vi "Einzelne Stufe aendern.vi"(4 "Component additional Index":i32[](array[numeric]), 5 "GD-Cluster":T3, 6 "Component GD Index":i32[](array[numeric]), 7 "GD LNI Cluster":T2, 8 "error in (no error)":errorcluster caption="Fehler (Eingang, kein Fehler)", 9 "Komponentenauswahl":T7 {"Konzentration" format="%#.6f"}, 10 "Zeile Punkt Änderung Cluster":cluster{"Zeile":i32, "Punkt":string}, 11 "Stufen Tabellen in":string[][][](array[string])) -> (0 "error out":errorcluster caption="Fehler (Ausgang)", 1 "Component Index out":i32, 2 "Komponente out":T6, 3 "GD out":T5)   [LabVIEW 2020, in "Linearisierung v2.lvlib" / "Gasteiler.lvlib"]
uses:
  Gasteiler.lvlib
  KomponentenArray.ctl
  Visualisierungs Elemente/Auswahlfeld.ctl
  Seiten/System Einstellungen V2/Traegergas.ctl
  Visualisierungs Elemente/Checkbox(boolsch).ctl
  Aktionen FGV Gasteiler Daten.ctl
  Aktion FGV Gasteilerliste laden.ctl
  AK-Komm Gasteiler/Aktionen AK Komm.ctl
  AK-Komm Gasteiler/Alter Gasteiler/Aktionen AK Komm_ALT.ctl
  Horiba/Aktion Befehl.ctl
  AK-Komm Gasteiler/AK Komm Gasteiler.lvlib
  Horiba/Horiba GDC.lvlib
  AK-Komm Gasteiler/Alter Gasteiler/Alter Gasteiler.lvlib
  Linearisierung v2.lvlib
  Aktion Lin Daten aufarbeiten.ctl
  Seiten/System Einstellungen V2/System Einstellungen V2.lvlib
  HovaCal/HovaCal.lvlib
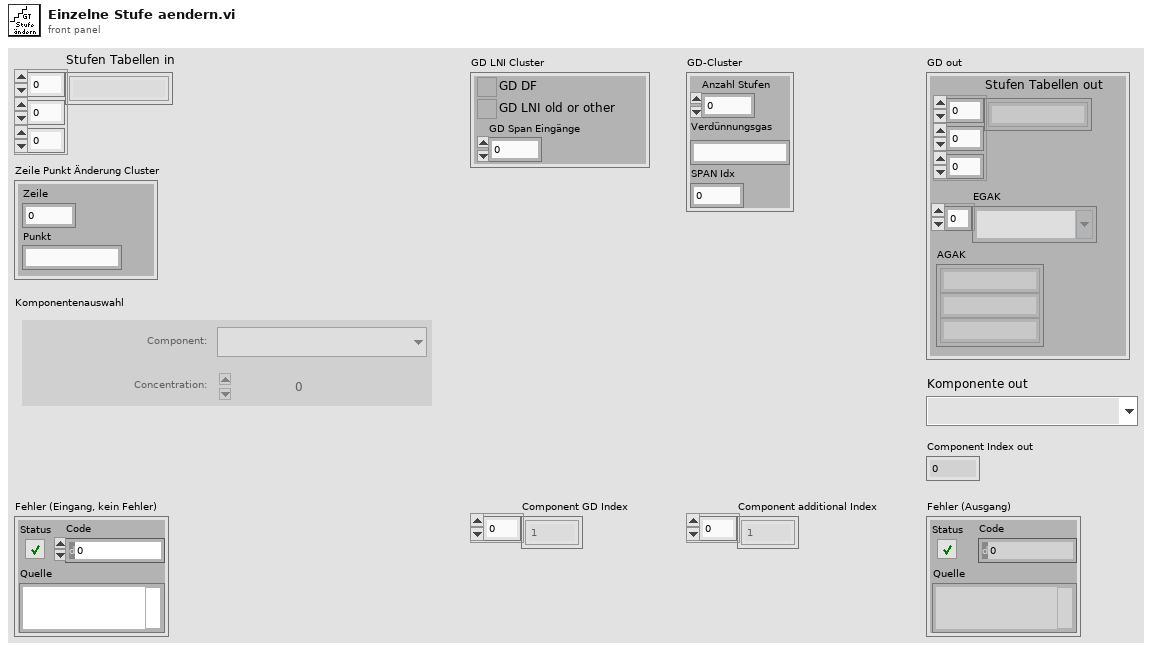
[diagram p1: front panel]
types:
  T1 = typedef "Checkbox(boolsch).ctl" = bool
  T2 = cluster{"GD DF":T1, "GD LNI old or other":T1, "GD Span Eingänge":u16}
  T3 = cluster{"Anzahl Stufen":sgl, "Verdünnungsgas":string, "SPAN Idx":i32}
  T4 = typedef "System Einstellungen V2.lvlib/Traegergas.ctl" = string
  T5 = cluster{"Stufen Tabellen out":string[][][], "EGAK":T4[], "AGAK":string[]}
  T6 = typedef "Auswahlfeld.ctl" = u16
  T7 = typedef "Linearisierung v2.lvlib/KomponentenArray.ctl" = cluster{"Komponente:":T6, "Konzentration":dbl}[]
  T8 = typedef "Linearisierung v2.lvlib/Gasteiler.lvlib/Aktionen FGV Gasteiler Daten.ctl" = enum16{"lesen", "Gasteiler Daten", "Seriellen Param.", "MB-Endwert", "laden", "speichern", "Anforderung", "TCP", "Aufzeichnung Start"}
  T9 = typedef "Linearisierung v2.lvlib/Aktion Lin Daten aufarbeiten.ctl" = enum16{"lesen", "Protkolldaten", "speichern", "laden", "EPA auswerten", "Tabelle schreiben", "Lin auswerten", "Tab init", "Stufentabelle", "EPA aktiviert", "Nachbehandlung laden", "Tabelle löschen", "Istwerte löschen", "Zeile löschen", "Zeile einfügen", "LIN aktiviert", "LIN/EPA aktiv laden", "EGAK Tab", "LIN übernehmen", "Tab init ohne Stufen"}
  T10 = typedef "Linearisierung v2.lvlib/Lin-Polynom Daten.ctl" = cluster{"Messgerät":string, "Kalibrator (Gasteiler)":string, "Bearbeiter/in":string, "Komponente":string, "Zeitstempel":timestamp, "F_max gefordert (%)":sgl, "F_max in %":sgl, "F_max in ppm":sgl, "Vorschlag Ordnung":i32, "Polynom OK":bool, "Polynomkoeff.":dbl[], "Prüfgas Konzentration":dbl, "Pfad EPA":string, "Pfad_LIN":string, "Gasnummer:":u8, "Komponentenauswahl":T7, "Verdünnungsgas":T11, "Zeitdauer Stufe":T12, "Anzahl Stufen":T12, "F_max in % EPA":sgl, "F_max in ppm EPA":sgl, "F_max in % LIN":sgl, "F_max in ppm LIN":sgl, "Punkte umkehren":bool, "EPA Optionsfeld":T13, "Autolin Hovacal":T14, "Spanfactors":sgl[], "Kalibrierauswahl":T15, "Conditions:":T16, "Gasflaschen Nr.:":string, "Bottle Accuracy":dbl, "Konfig Gasflasche":T17, "Gasflasche":T18, "HovaCAL Flow AutoLin":T19, "MFC Output":T20, "Gas Ablaufdatum":timestamp, "Lin Modus":T21, "zusätzliche Zeitdauer Erster Punkt":sgl, "Offsets":sgl[]}
  T11 = typedef "Linearisierung v2.lvlib/Gasteiler.lvlib/Prüfgas in.ctl" = u16
  T12 = typedef "Zahlen-Eingabefeld.ctl" = sgl
  T13 = typedef "Linearisierung v2.lvlib/EPA Optionsfeld.ctl" = enum32{"Istwert", "Rohwert", "Linearisierter Wert"}
  T14 = typedef "Linearisierung v2.lvlib/Gasteiler.lvlib/HovaCal.lvlib/AutoLin Hovacal.ctl" = enum32{"Keine Auswahl", "Optionsauswahl 1", "Optionsauswahl 2"}
  T15 = typedef "Linearisierung v2.lvlib/Kalibrieroption.ctl" = u16
  T16 = typedef "Linearisierung v2.lvlib/Linearity verification 1065-307.lvlib/Condition.ctl" = u16
  T17 = typedef "System Einstellungen V2.lvlib/Konfig Gasflasche.ctl" = bool
  T18 = typedef "System Einstellungen V2.lvlib/Gasflasche Auswahl.ctl" = u16
  T19 = typedef "Linearisierung v2.lvlib/Gasteiler.lvlib/HovaCAL_Interface.lvlib/Controls.lvlib/Flow Einstellung.ctl" = cluster{"HovaCAL Flow Input Cluster":dbl}
  T20 = typedef "Linearisierung v2.lvlib/Gasteiler.lvlib/HovaCAL_Interface.lvlib/Controls.lvlib/Pump state.ctl" = cluster{"Run":bool}
  T21 = typedef "Linearisierung v2.lvlib/Lin Modus.ctl" = u16
  T22 = typedef "Linearisierung v2.lvlib/Gasteiler.lvlib/Aktion FGV Gasteilerliste laden.ctl" = enum16{"lesen", "laden", "speichern", "Liste erstellen", "Formel ändern", "Gas vereinzeln"}
  T23 = typedef "Linearisierung v2.lvlib/Gasteiler.lvlib/Gasteiler Daten.ctl" = cluster{"Gasteiler":T24, "Gasteiler Stufen":T25, "Gasteiler Type":T26, "Konfig Gasteiler":T27, "Gasteiler Span Eingänge":u16}
  T24 = typedef "String - Eingabefeld.ctl" = string
  T25 = typedef "Linearisierung v2.lvlib/Gasteiler.lvlib/Gasteiler Stufen.ctl" = u16
  T26 = typedef "Linearisierung v2.lvlib/GasteilerType.ctl" = u16
  T27 = typedef "System Einstellungen V2.lvlib/Gasteiler Auswahl.ctl" = u16
  T28 = typedef "Linearisierung v2.lvlib/Gasteiler.lvlib/AK Komm Gasteiler.lvlib/Aktionen AK Komm.ctl" = enum16{"lesen", "initialisieren", "beenden", "Status", "SMAN", "SREM", "STBY", "ASTF", "ASTZ", "SLST", "AGAT", "EGAK", "AGAK", "AKAK", "ADRU", "SKOP", "SVSA", "SVSZ", "SONO", "SAIR", "SNOX", "ANOX", "SSPL", "SRUC", "SLIN", "ALST", "ETYP", "SVIO", "LCYL", "CCYL", "DCYL", "SCYL", "GCYL", "DRGV", "DRDC"}
  T29 = typedef "Linearisierung v2.lvlib/Gasteiler.lvlib/AK Komm Gasteiler.lvlib/Alter Gasteiler.lvlib/Aktionen AK Komm_ALT.ctl" = enum16{"lesen", "initialisieren", "beenden", "SRES", "STBY", "SREM", "SMAN", "SLIN", "SLCH", "SLST", "SSPL", "AGAT", "ALST", "ASTZ", "ASTF", "AGAK", "EGAK"}
  T30 = typedef "Linearisierung v2.lvlib/Gasteiler.lvlib/Horiba GDC.lvlib/Aktion Befehl.ctl" = enum16{"lesen", "initialisieren", "Beenden", "Standby", "GD/CC", "Info", "Flow", "Alarm", "GD parameter", "GD point", "Durchfluss", "Spuelen1", "Spuelen1 On", "Spuelen1Off", "Spuelen2", "Ventil-Abfrage", "Reset"}
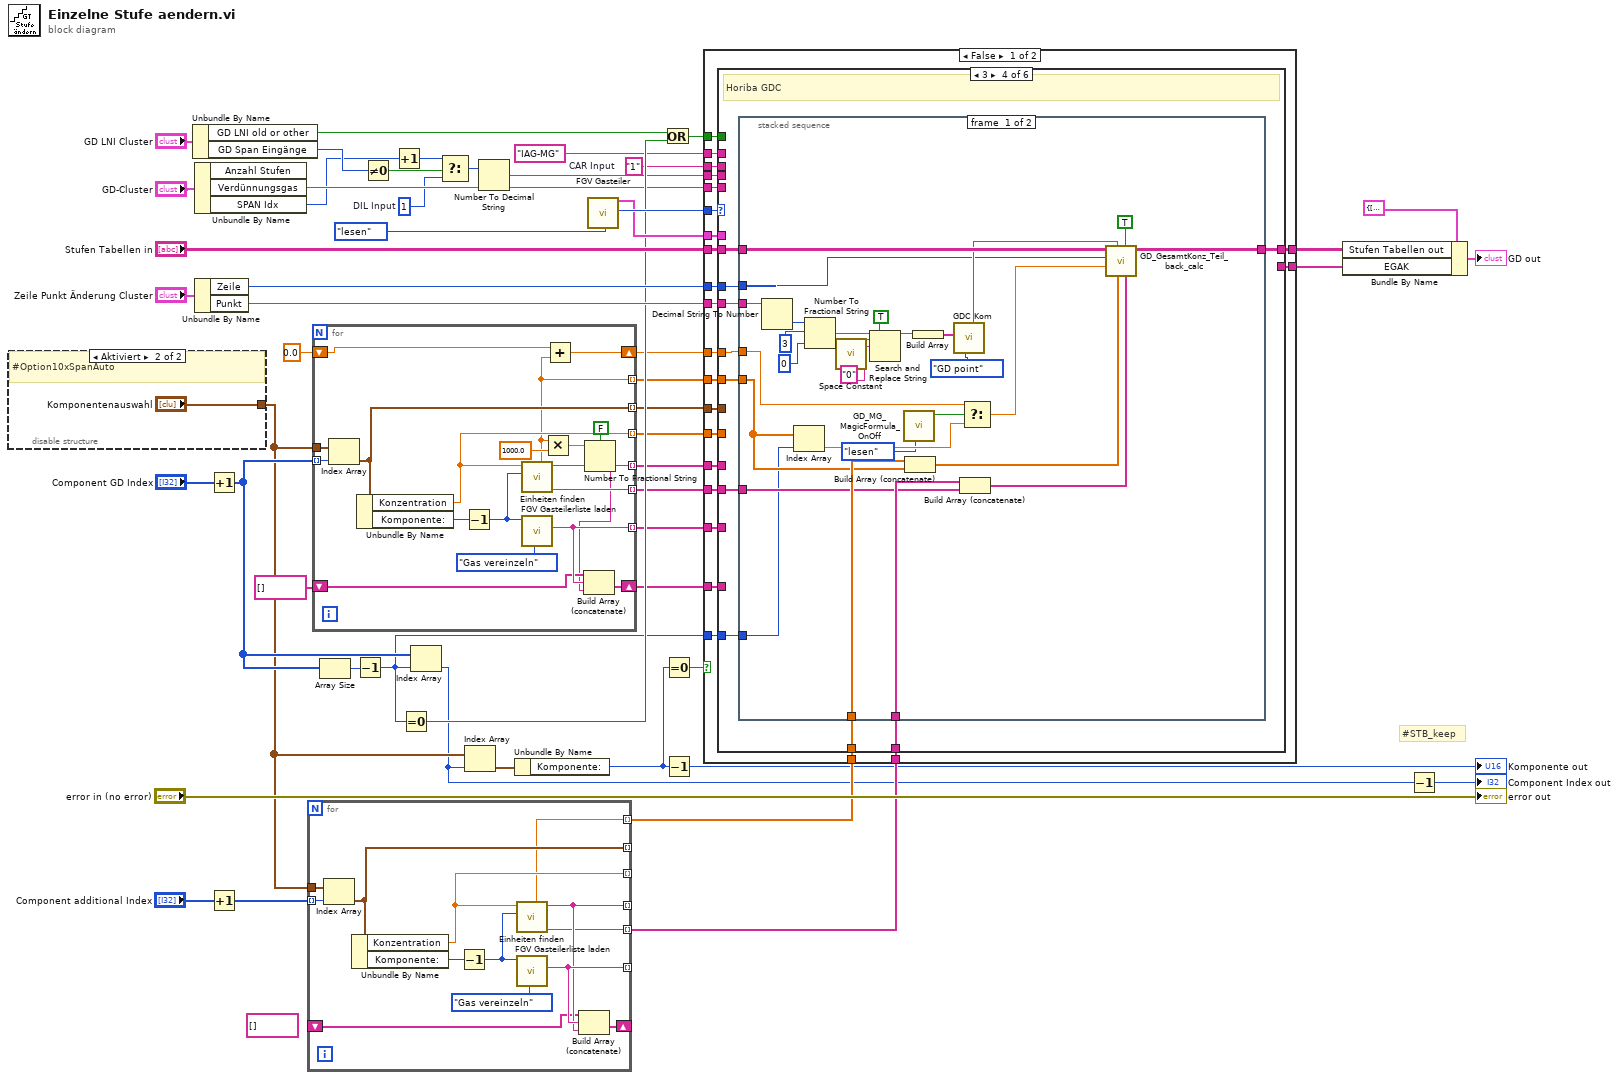
[diagram p0: block diagram]
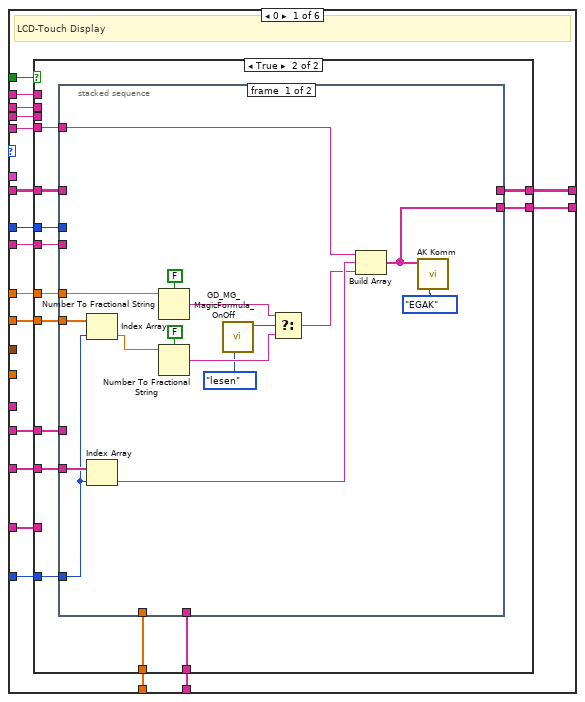
[diagram p2: hidden frame]
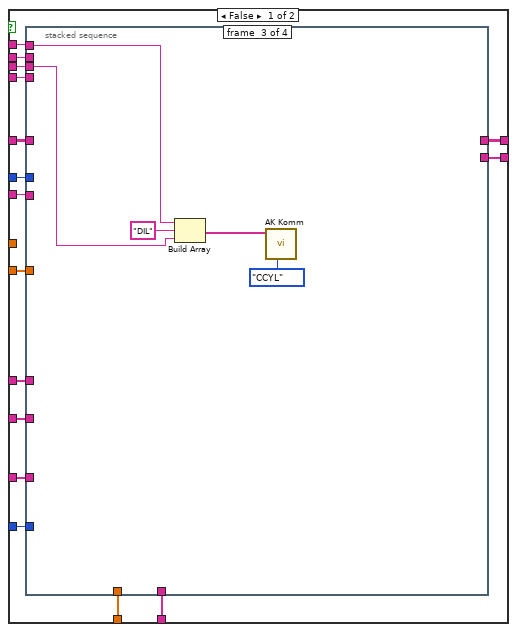
[diagram p3: hidden frame]
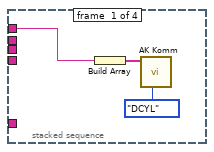
[diagram p4: hidden frame]
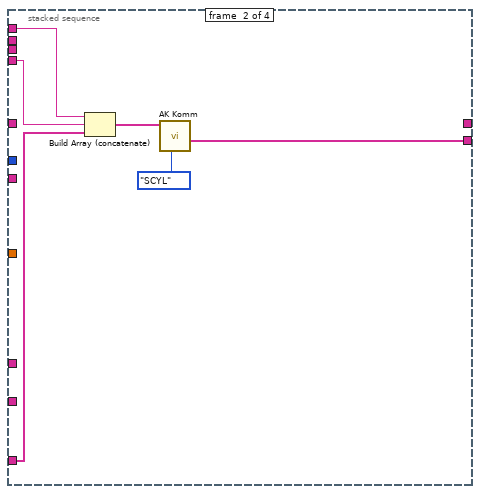
[diagram p5: hidden frame]
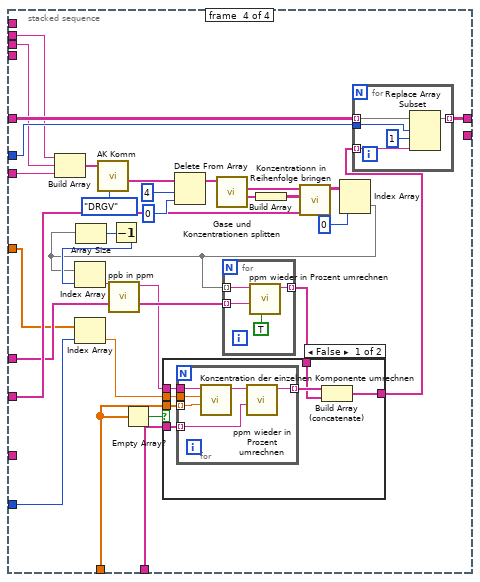
[diagram p6: hidden frame]
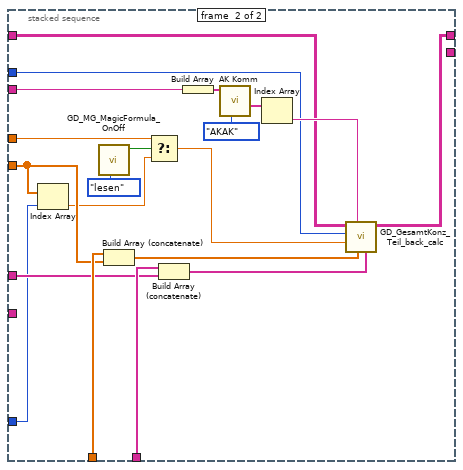
[diagram p8: hidden frame]
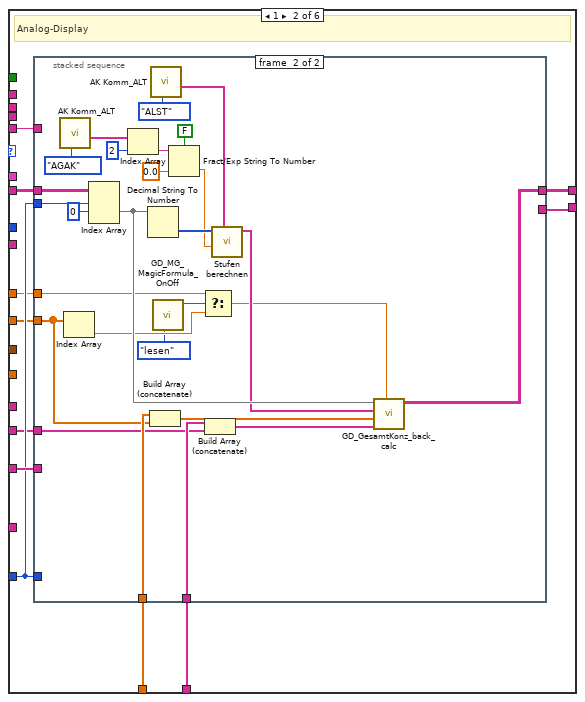
[diagram p9: hidden frame]
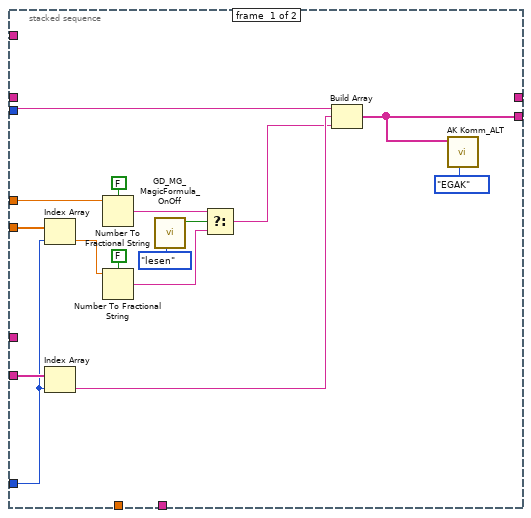
[diagram p10: hidden frame]
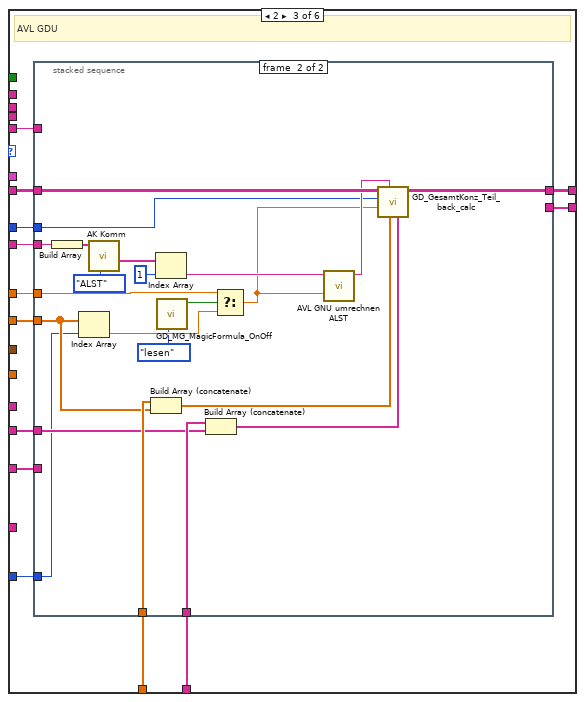
[diagram p11: hidden frame]
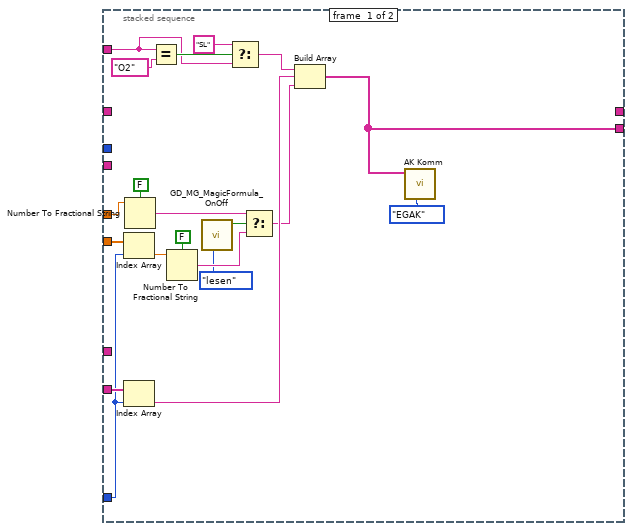
[diagram p12: hidden frame]
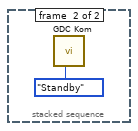
[diagram p13: hidden frame]
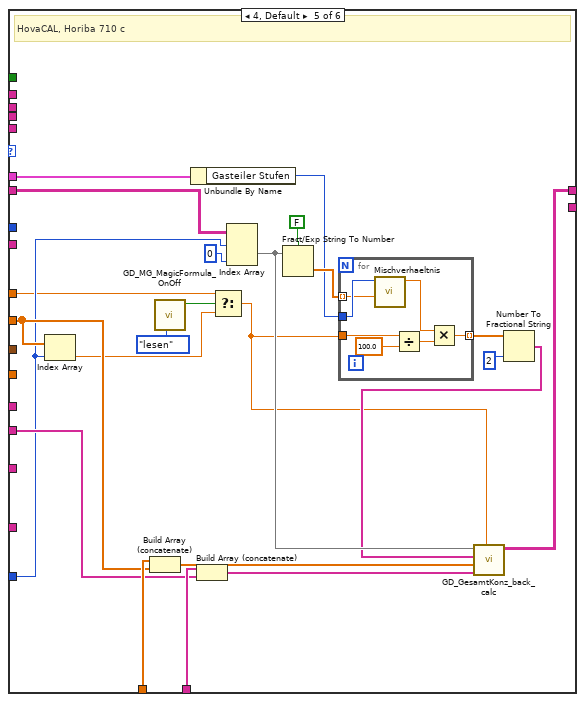
[diagram p14: hidden frame]
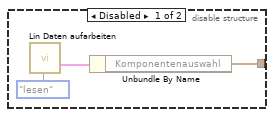
[diagram p17: hidden frame]
diagram:
  w10 = 1  # DIL Input
  w14 = "1"  # CAR Input
  (unwired) string[] []
  # "#STB_keep"
  n1 = disable-structure shown="Aktiviert" {
    disable-tunnel: [w53 "Komponentenauswahl"] -> w24
    frame Disabled {
      n2 = call "Lin Daten aufarbeiten.vi"("Aktionen"=Aktion_Lin_Daten_aufarbeiten."lesen") -> ("Lin-Polynom"=w54:T10)  [unwired: 16 in, 10 out]
      n3 = Unbundle By Name(w54) -> ("Komponentenauswahl"=w53:T7)
    }
    frame Enabled {
      # "#Option10xSpanAuto"
    }
  }
  n4 = Unbundle By Name("GD LNI Cluster") -> ("GD LNI old or other"=w12:T1, "GD Span Eingänge"=w8:u16)
  n5 = Unbundle By Name("GD-Cluster") -> ("Verdünnungsgas"=w27:string, "SPAN Idx"=w7:i32)  [unwired: 1 out]
  n6 = Unbundle By Name("Zeile Punkt Änderung Cluster") -> ("Zeile"=w44:i32, "Punkt"=w43:string)
  n7 = Increment(x="Component GD Index") -> (x+1=w36:i32[])
  n8 = Increment(x="Component additional Index") -> (x+1=w25:i32[])
  n9 = for {
    tunnel: w24 -> [w69]
    tunnel: w25 -> [w68] mode=indexing
    tunnel: [w63] -> _ mode=indexing
    tunnel: [w64] -> _ mode=indexing
    shift-right: [w62] -> _
    shift-left: _ -> [w61]
    tunnel: [w60] -> w22 mode=indexing
    tunnel: [w59] -> _ mode=indexing
    tunnel: [w58] -> _ mode=indexing
    tunnel: [w57] -> w23 mode=indexing
    n10 = Index Array(array=w69, index=w68) -> (element=w58:cluster{"Komponente:":T6, "Konzentration":dbl})
    n11 = Unbundle By Name(w58) -> ("Konzentration"=w59:dbl, "Komponente:"=w66:T6)
    n12 = Decrement(x=w66) -> (x-1=w65:T6)
    n13 = call "Einheiten finden.vi"("Komponente"=w65, "Wert"=w59) -> ("Einheit in String"=w60:string, "String"=w63:string, "Wert ppm"=w57:dbl)  [unwired: 5 in, 2 out]
    n14 = call "FGV Gasteilerliste laden.vi"("Aktion"=Aktion_FGV_Gasteilerliste_laden."Gas vereinzeln", "Gasindex"=w65) -> ("Formel"=w64:string)  [unwired: 7 in, 2 out]
    n15 = Build Array (concatenate)(w61, w64, w63) -> (w62:string[])
  }
  n16 = for {
    tunnel: w24 -> [w88]
    tunnel: w36 -> [w87] mode=indexing
    tunnel: [w82] -> w16 mode=indexing
    tunnel: [w83] -> w21 mode=indexing
    shift-right: [w81] -> w26
    shift-left: string[] [] -> [w80]
    tunnel: [w79] -> w15 mode=indexing
    tunnel: [w78] -> w17 mode=indexing
    tunnel: [w77] -> w20 mode=indexing
    shift-right: [w76] -> w19
    shift-left: 0.0 -> [w75]
    tunnel: [w71] -> w18 mode=indexing
    n17 = Index Array(array=w88, index=w87) -> (element=w77:cluster{"Komponente:":T6, "Konzentration":dbl})
    n18 = Unbundle By Name(w77) -> ("Konzentration"=w78:dbl, "Komponente:"=w85:T6)
    n19 = Decrement(x=w85) -> (x-1=w84:T6)
    n20 = call "Einheiten finden.vi"("Komponente"=w84, "Wert"=w78) -> ("Einheit in String"=w79:string, "String"=w82:string, "Wert ppm"=w71:dbl)  [unwired: 5 in, 2 out]
    n21 = call "FGV Gasteilerliste laden.vi"("Aktion"=Aktion_FGV_Gasteilerliste_laden."Gas vereinzeln", "Gasindex"=w84) -> ("Formel"=w83:string)  [unwired: 7 in, 2 out]
    n22 = Multiply(x=w71, y=1000.0) -> (x*y=w73:dbl)
    n23 = Add(x=w75, y=w71) -> (x+y=w76:dbl)
    n24 = Number To Fractional String(use system decimal point (T)=FALSE ("Systemdezimalzeichen verwenden (T)"), number=w73) -> (F-format string=w70:string)  [unwired: 2 in]
    n25 = Build Array (concatenate)(w80, w83, w70) -> (w81:string[])
  }
  n26 = Array Size(array=w36) -> (size(s)=w2:i32)
  n27 = Decrement(x=w2) -> (x-1=w33:i32)
  n28 = Not Equal To 0?(x=w8) -> (x != 0?=w11:bool)
  n29 = Increment(x=w7) -> (x+1=w9:i32)
  n30 = Equal To 0?(x=w33) -> (x = 0?=w34:bool)
  n31 = Index Array(array=w36, index=w33) -> (element=w3:i32)
  n32 = Select(t=w9, s=w11, f=w10) -> (s? t:f=w6:i32)
  n33 = Index Array(array=w24, index=w3) -> (element=w32:cluster{"Komponente:":T6, "Konzentration":dbl})
  n34 = Number To Decimal String(number=w6) -> (decimal integer string=w5:string)  [unwired: 1 in]
  n35 = Unbundle By Name(w32) -> ("Komponente:"=w31:T6)
  n36 = call "FGV Gasteiler.vi"("Aktionen"=Aktionen_FGV_Gasteiler_Daten."lesen") -> ("Gasteiler Daten"=w46:T23, "Gasteiler Type"=w52:T26)  [unwired: 11 in, 6 out]
  n37 = Or(x=w12, y=w34) -> (x .or. y?=w29:T1)
  n38 = Equal To 0?(x=w31) -> (x = 0?=w35:bool)
  n39 = Decrement(x=w31) -> (x-1=→"Komponente out":T6)
  n40 = case shown="False" w35 {
    tunnel: w52 -> [w111 _]
    tunnel: "Stufen Tabellen in" -> [w110 w443]
    tunnel: w44 -> [w109 _]
    tunnel: w43 -> [w108 _]
    tunnel: [w107 w443] -> w49
    tunnel: [w106 _] -> w48
    tunnel: w20 -> [w105 _]
    tunnel: w46 -> [w104 _]
    tunnel: w33 -> [w103 _]
    tunnel: "IAG-MG" -> [w102 _]
    tunnel: w29 -> [w101 _]
    tunnel: w27 -> [w100 _]
    tunnel: w26 -> [w99 _]
    tunnel: w23 -> [w98 _]
    tunnel: w22 -> [w97 _]
    tunnel: w21 -> [w96 _]
    tunnel: w19 -> [w95 _]
    tunnel: w18 -> [w93 _]
    tunnel: w17 -> [w94 _]
    tunnel: w16 -> [w92 _]
    tunnel: w15 -> [w91 _]
    tunnel: w14 -> [w90 _]
    tunnel: w5 -> [w89 _]
    frame False {
      n41 = case shown="3" w111 {
        tunnel: w110 -> [w117 w272 w326 w382 w434 w442]
        tunnel: [w129 w274 w330 w381 w419 w442] -> w107
        tunnel: w109 -> [w128 _ w328 w379 _ _]
        tunnel: w108 -> [w127 _ w329 w380 _ _]
        tunnel: [w126 w273 w327 _ _ _] -> w106
        tunnel: w105 -> [_ _ _ _ _ _]
        tunnel: w104 -> [_ _ _ _ w431 _]
        tunnel: w103 -> [w115 w269 w323 w373 w417 _]
        tunnel: w102 -> [w124 _ _ _ _ _]
        tunnel: w101 -> [w125 _ _ _ _ _]
        tunnel: w100 -> [w123 w271 w325 _ _ _]
        tunnel: w99 -> [w122 _ _ _ _ _]
        tunnel: w98 -> [w120 w267 w321 w378 w427 _]
        tunnel: w97 -> [w119 w266 w320 w377 w426 _]
        tunnel: w96 -> [w116 w270 w324 _ _ _]
        tunnel: w95 -> [w121 w264 w322 w376 w416 _]
        tunnel: w94 -> [_ _ _ _ _ _]
        tunnel: w93 -> [w114 w268 w318 w375 w418 _]
        tunnel: w92 -> [_ _ _ _ _ _]
        tunnel: w91 -> [w118 w265 w319 w374 w425 _]
        tunnel: w90 -> [w113 _ _ _ _ _]
        tunnel: w89 -> [w112 _ _ _ _ _]
        frame 0 {
          # "LCD-Touch Display"
          n42 = case shown="True" w125 {
            tunnel: [w132 w227] -> w129
            tunnel: w128 -> [w136 w226]
            tunnel: w127 -> [w141 w225]
            tunnel: [w142 w224] -> w126
            tunnel: w117 -> [w137 w223]
            tunnel: w124 -> [w145 _]
            tunnel: w123 -> [w144 w222]
            tunnel: w122 -> [w143 _]
            tunnel: w121 -> [_ w218]
            tunnel: w120 -> [w134 w221]
            tunnel: w119 -> [w133 w220]
            tunnel: w118 -> [w139 w219]
            tunnel: w116 -> [w140 w216]
            tunnel: w115 -> [w138 w215]
            tunnel: w114 -> [w135 w217]
            tunnel: w113 -> [w131 _]
            tunnel: w112 -> [w130 _]
            frame False {
              n43 = stacked-sequence {
                tunnel: w145 -> [w146 w152 w156 _]
                tunnel: w144 -> [_ w151 _ _]
                tunnel: w143 -> [_ w150 _ _]
                tunnel: w141 -> [_ _ _ w185]
                tunnel: [_ w149 _ _] -> w142
                tunnel: w140 -> [_ _ _ w184]
                tunnel: w139 -> [_ _ _ w180]
                tunnel: w138 -> [_ _ _ w164]
                tunnel: w137 -> [_ _ _ w175]
                tunnel: w136 -> [_ _ _ w176]
                tunnel: w135 -> [_ _ _ w179]
                tunnel: w134 -> [_ _ _ w168]
                tunnel: w133 -> [_ _ _ w177]
                tunnel: [_ _ _ w173] -> w132
                tunnel: w131 -> [_ _ _ w171]
                tunnel: w130 -> [_ _ w155 w170]
                frame #0 {
                  n44 = Build Array(w146) -> (w147:string[])
                  n45 = call "AK Komm.vi"("Aktionen"=Aktionen_AK_Komm."DCYL", "Daten"=w147) -> ()  [unwired: 3 in, 7 out]
                }
                frame #1 {
                  n46 = Build Array (concatenate)(w152, w151, w150) -> (w153:string[])
                  n47 = call "AK Komm.vi"("Aktionen"=Aktionen_AK_Komm."SCYL", "Daten"=w153) -> ("Empfangsdaten"=w149:string[])  [unwired: 3 in, 6 out]
                }
                frame #2 {
                  n48 = Build Array(w156, "DIL", w155) -> (w158:string[])
                  n49 = call "AK Komm.vi"("Aktionen"=Aktionen_AK_Komm."CCYL", "Daten"=w158) -> ()  [unwired: 3 in, 7 out]
                }
                frame #3 {
                  n50 = Build Array(w171, w170, w185) -> (w190:string[])
                  n51 = Index Array(array=w179, index=w164) -> (element=w178:dbl)
                  n52 = call "AK Komm.vi"("Aktionen"=Aktionen_AK_Komm."DRGV", "Daten"=w190) -> ("Empfangsdaten"=w189:string[])  [unwired: 3 in, 6 out]
                  n53 = Empty Array?(array=w168) -> (empty?=w169:bool)
                  n54 = Delete From Array(array=w189, length=4 ("Länge"), index=0 ("Index")) -> (array with subset deleted=w186:string[])  [unwired: 1 out]
                  n55 = call "Gase und Konzentrationen splitten.vi"("Empfangsdaten (Eingang)"=w186) -> ("Konzentrationen"=w183:string[], "Gase"=w166:string[])  [unwired: 9 in]
                  n56 = Build Array(w183) -> (w182:string[][])
                  n57 = call "Konzentrationn in Reihenfolge bringen.vi"("Gas Namen"=w184, "Konzentrationen"=w182, "Gase"=w166) -> ("Stufen ja Gas"=w181:string[][])  [unwired: 8 in]
                  n58 = Index Array(array=w181, index (col)=0 ("Deaktivierter Index (Spalte)")) -> (element=w163:string[])  [unwired: 1 in]
                  n59 = Array Size(array=w163) -> (size(s)=w167:i32)
                  n60 = Decrement(x=w167) -> (x-1=w165:i32)
                  n61 = Index Array(array=w163, index=w165) -> (element=w161:string)
                  n62 = call "ppb in ppm.vi"("Werteingang"=w161) -> ("Wertausgang"=w160:string)  [unwired: 9 in]
                  n63 = for {
                    tunnel: w180 -> [w214] mode=indexing
                    tunnel: [w213] -> w174 mode=indexing
                    tunnel: w163 -> [w212] mode=indexing
                    n64 = call "ppm wieder in Prozent umrechnen.vi"("LNI_ppb"=TRUE, "Einheit"=w214, "Werteingang"=w212) -> ("Wertausgang"=w213:string)  [unwired: 8 in]
                  }
                  n65 = case shown="False" w169 {
                    tunnel: w160 -> [w198 _]
                    tunnel: w178 -> [w197 _]
                    tunnel: w168 -> [w196 _]
                    tunnel: w177 -> [w195 _]
                    tunnel: w174 -> [w193 w205]
                    tunnel: [w192 w205] -> w172
                    frame False {
                      n66 = for {
                        tunnel: w196 -> [w202] mode=indexing
                        tunnel: w195 -> [w201] mode=indexing
                        tunnel: w198 -> [w203]
                        tunnel: w197 -> [w200]
                        tunnel: [w199] -> w194 mode=indexing
                        n67 = call "Konzentration der einzelnen Komponente umrechnen.vi"("Teilkonzentration"=w202, "Gesamtkonzentration"=w200, "Werteingang"=w203) -> ("Wertausgang"=w204:string)  [unwired: 8 in]
                        n68 = call "ppm wieder in Prozent umrechnen.vi"("Einheit"=w201, "Werteingang"=w204) -> ("Wertausgang"=w199:string)  [unwired: 9 in]
                      }
                      n69 = Build Array (concatenate)(w194, w193) -> (w192:string[])
                    }
                    frame True {
                    }
                  }
                  n70 = for {
                    tunnel: w176 -> [w209]
                    tunnel: w175 -> [w208] mode=indexing
                    tunnel: [w207] -> w173 mode=indexing
                    tunnel: w172 -> [w206] mode=indexing
                    n71 = Replace Array Subset(array=w208, new element=w206, index (row)=w209, index (col)=1 ("Deaktivierter Index (Spalte)")) -> (w207:string[][])
                  }
                }
              }
            }
            frame True {
              n72 = stacked-sequence {
                tunnel: w223 -> [_ w252]
                tunnel: [_ w251] -> w227
                tunnel: w226 -> [_ w253]
                tunnel: w225 -> [_ w260]
                tunnel: [w241 _] -> w224
                tunnel: w222 -> [w242 _]
                tunnel: w221 -> [_ w259]
                tunnel: w220 -> [_ w258]
                tunnel: w219 -> [_ w257]
                tunnel: w218 -> [w240 w246]
                tunnel: w217 -> [w236 w249]
                tunnel: w216 -> [w238 _]
                tunnel: w215 -> [w235 w248]
                frame #0 {
                  n73 = Index Array(array=w236, index=w235) -> (element=w233:dbl)
                  n74 = Index Array(array=w238, index=w235) -> (element=w237:string)
                  n75 = Number To Fractional String(use system decimal point (T)=FALSE ("Systemdezimalzeichen verwenden (T)"), number=w240) -> (F-format string=w229:string)  [unwired: 2 in]
                  n76 = Number To Fractional String(use system decimal point (T)=FALSE ("Systemdezimalzeichen verwenden (T)"), number=w233) -> (F-format string=w231:string)  [unwired: 2 in]
                  n77 = call "GD_MG_MagicFormula_OnOff.vi"("Aktion"=enum16{"lesen", "schreiben", "init"}."lesen") -> ("MG_use_magic_formula"=w232:bool)  [unwired: 8 in, 1 out]
                  n78 = Select(t=w229, s=w232, f=w231) -> (s? t:f=w230:string)
                  n79 = Build Array(w242, w237, w230) -> (w241:string[])
                  n80 = call "AK Komm.vi"("Aktionen"=Aktionen_AK_Komm."EGAK", "Daten"=w241) -> ()  [unwired: 3 in, 7 out]
                }
                frame #1 {
                  n81 = Index Array(array=w249, index=w248) -> (element=w247:dbl)
                  n82 = call "GD_MG_MagicFormula_OnOff.vi"("Aktion"=enum16{"lesen", "schreiben", "init"}."lesen") -> ("MG_use_magic_formula"=w250:bool)  [unwired: 8 in, 1 out]
                  n83 = Build Array (concatenate)(w259, w249) -> (w256:dbl[])
                  n84 = Select(t=w246, s=w250, f=w247) -> (s? t:f=w245:dbl)
                  n85 = Build Array (concatenate)(w258, w257) -> (w255:string[])
                  n86 = Build Array(w260) -> (w262:string[])
                  n87 = call "AK Komm.vi"("Aktionen"=Aktionen_AK_Komm."AKAK", "Daten"=w262) -> ("Empfangsdaten"=w261:string[])  [unwired: 3 in, 6 out]
                  n88 = Index Array(array=w261) -> (element=w254:string)  [unwired: 1 in]
                  n89 = call "GD_GesamtKonz_Teil_back_calc.vi"("Einheiten"=w255, "Konzentration der Komponenten"=w256, "Stufen"=w254, "Gesamtkonzentration"=w245, "Zeile"=w253, "Stufen Tabellen in (Eingang)"=w252) -> ("Stufen Tabellen in (Ausgang)"=w251:string[][][])  [unwired: 5 in]
                }
              }
            }
          }
        }
        frame 1 {
          # "Analog-Display"
          n90 = stacked-sequence {
            tunnel: w272 -> [_ w315]
            tunnel: [_ w297] -> w274
            tunnel: [w288 _] -> w273
            tunnel: w271 -> [w289 _]
            tunnel: w269 -> [_ w305]
            tunnel: w270 -> [w287 _]
            tunnel: w269 -> [w281 _]
            tunnel: w268 -> [w282 w294]
            tunnel: w267 -> [_ w304]
            tunnel: w266 -> [_ w303]
            tunnel: w265 -> [_ w302]
            tunnel: w264 -> [w285 w293]
            frame #0 {
              n91 = Index Array(array=w282, index=w281) -> (element=w279:dbl)
              n92 = Index Array(array=w287, index=w281) -> (element=w286:string)
              n93 = Number To Fractional String(use system decimal point (T)=FALSE ("Systemdezimalzeichen verwenden (T)"), number=w285) -> (F-format string=w277:string)  [unwired: 2 in]
              n94 = Number To Fractional String(use system decimal point (T)=FALSE ("Systemdezimalzeichen verwenden (T)"), number=w279) -> (F-format string=w278:string)  [unwired: 2 in]
              n95 = call "GD_MG_MagicFormula_OnOff.vi"("Aktion"=enum16{"lesen", "schreiben", "init"}."lesen") -> ("MG_use_magic_formula"=w283:bool)  [unwired: 8 in, 1 out]
              n96 = Select(t=w277, s=w283, f=w278) -> (s? t:f=w276:string)
              n97 = Build Array(w289, w286, w276) -> (w288:string[])
              n98 = call "AK Komm_ALT.vi"("Aktionen_ALT"=Aktionen_AK_Komm_ALT."EGAK", "Daten"=w288) -> ()  [unwired: 5 in, 5 out]
            }
            frame #1 {
              n99 = call "AK Komm_ALT.vi"("Aktionen_ALT"=Aktionen_AK_Komm_ALT."AGAK") -> ("Empfangsdaten"=w308:string[])  [unwired: 6 in, 4 out]
              n100 = Index Array(array=w294) -> (element=w295:dbl)  [unwired: 1 in]
              n101 = Index Array(array=w315, index (dim 0)=w305, index (dim 1)=0 ("Deaktivierter Index (Spalte)")) -> (element=w301:string[])  [unwired: 1 in]
              n102 = Index Array(array=w308, index=2 ("Index")) -> (element=w311:string)
              n103 = Decimal String To Number(string=w301) -> (number=w313:i32[])  [unwired: 2 in, 1 out]
              n104 = Build Array (concatenate)(w304, w294) -> (w299:dbl[])
              n105 = call "AK Komm_ALT.vi"("Aktionen_ALT"=Aktionen_AK_Komm_ALT."ALST") -> ("Empfangsdaten"=w316:string[])  [unwired: 6 in, 4 out]
              n106 = call "GD_MG_MagicFormula_OnOff.vi"("Aktion"=enum16{"lesen", "schreiben", "init"}."lesen") -> ("MG_use_magic_formula"=w296:bool)  [unwired: 8 in, 1 out]
              n107 = Fract/Exp String To Number(use system decimal point (T)=FALSE ("Systemdezimalzeichen verwenden (T)"), string=w311, default (0 dbl)=sgl 0.0 ("Standard (0 DBL)")) -> (number=w306:sgl)  [unwired: 1 in, 1 out]
              n108 = Select(t=w293, s=w296, f=w295) -> (s? t:f=w292:dbl)
              n109 = Build Array (concatenate)(w303, w302) -> (w298:string[])
              n110 = call "Stufen berechnen.vi"("Empfangsdaten"=w316, "Konzentration"=w306, "Stufen"=w313) -> ("Stufen Tabelle"=w300:string[])  [unwired: 7 in, 1 out]
              n111 = call "GD_GesamtKonz_back_calc.vi"("Gesamtkonzentration"=w292, "Einheiten"=w298, "Konzentration der Komponenten"=w299, "Stufen"=w300, "Punkte (Eingang)"=w301) -> ("Stufentabellen (Ausgang)"=w297:string[][][])  [unwired: 5 in, 1 out]
            }
          }
        }
        frame 2 {
          # "AVL GDU"
          n112 = stacked-sequence {
            tunnel: w326 -> [_ w363]
            tunnel: [_ w362] -> w330
            tunnel: w328 -> [_ w360]
            tunnel: w329 -> [_ w369]
            tunnel: [w342 _] -> w327
            tunnel: w325 -> [w346 _]
            tunnel: w324 -> [w344 _]
            tunnel: w323 -> [w340 w354]
            tunnel: w322 -> [w333 w353]
            tunnel: w321 -> [_ w366]
            tunnel: w320 -> [_ w365]
            tunnel: w319 -> [_ w364]
            tunnel: w318 -> [w341 w355]
            frame #0 {
              n113 = Index Array(array=w341, index=w340) -> (element=w339:dbl)
              n114 = Index Array(array=w344, index=w340) -> (element=w343:string)
              n115 = Number To Fractional String(use system decimal point (T)=FALSE ("Systemdezimalzeichen verwenden (T)"), number=w333) -> (F-format string=w332:string)  [unwired: 2 in]
              n116 = Equal?(x=w346, y=T4 "O2") -> (x = y?=w348:bool)
              n117 = Number To Fractional String(use system decimal point (T)=FALSE ("Systemdezimalzeichen verwenden (T)"), number=w339) -> (F-format string=w336:string)  [unwired: 2 in]
              n118 = call "GD_MG_MagicFormula_OnOff.vi"("Aktion"=enum16{"lesen", "schreiben", "init"}."lesen") -> ("MG_use_magic_formula"=w337:bool)  [unwired: 8 in, 1 out]
              n119 = Select(t="SL" ("Formel"), s=w348, f=w346) -> (s? t:f=w345:string)
              n120 = Select(t=w332, s=w337, f=w336) -> (s? t:f=w335:string)
              n121 = Build Array(w345, w343, w335) -> (w342:string[])
              n122 = call "AK Komm.vi"("Aktionen"=Aktionen_AK_Komm."EGAK", "Daten"=w342) -> ()  [unwired: 3 in, 7 out]
            }
            frame #1 {
              n123 = Build Array(w369) -> (w371:string[])
              n124 = Index Array(array=w355, index=w354) -> (element=w356:dbl)
              n125 = call "AK Komm.vi"("Aktionen"=Aktionen_AK_Komm."ALST", "Daten"=w371) -> ("Empfangsdaten"=w370:string[])  [unwired: 3 in, 6 out]
              n126 = Build Array (concatenate)(w366, w355) -> (w358:dbl[])
              n127 = Index Array(array=w370, index=1 ("Deaktivierter Index (Spalte)")) -> (element=w368:string)
              n128 = call "GD_MG_MagicFormula_OnOff.vi"("Aktion"=enum16{"lesen", "schreiben", "init"}."lesen") -> ("MG_use_magic_formula"=w357:bool)  [unwired: 8 in, 1 out]
              n129 = Build Array (concatenate)(w365, w364) -> (w359:string[])
              n130 = Select(t=w353, s=w357, f=w356) -> (s? t:f=w352:dbl)
              n131 = call "AVL GNU umrechnen ALST.vi"("Konzentration"=w352, "Teilerstufe in%"=w368) -> ("Konzentration"=w361:string)  [unwired: 9 in]
              n132 = call "GD_GesamtKonz_Teil_back_calc.vi"("Einheiten"=w359, "Konzentration der Komponenten"=w358, "Stufen"=w361, "Gesamtkonzentration"=w352, "Zeile"=w360, "Stufen Tabellen in (Eingang)"=w363) -> ("Stufen Tabellen in (Ausgang)"=w362:string[][][])  [unwired: 5 in]
            }
          }
        }
        frame 3 {
          # "Horiba GDC"
          n133 = stacked-sequence {
            tunnel: w382 -> [w395 _]
            tunnel: [w394 _] -> w381
            tunnel: w380 -> [w400 _]
            tunnel: w379 -> [w392 _]
            tunnel: w378 -> [w399 _]
            tunnel: w377 -> [w398 _]
            tunnel: w376 -> [w385 _]
            tunnel: w375 -> [w387 _]
            tunnel: w374 -> [w397 _]
            tunnel: w373 -> [w386 _]
            frame #0 {
              n134 = Decimal String To Number(string=w400) -> (number=w410:i32)  [unwired: 2 in, 1 out]
              n135 = Index Array(array=w387, index=w386) -> (element=w388:dbl)
              n136 = Number To Fractional String(number=w410, width (-)=i16 3 ("Breite (-)"), precision (6)=i16 0 ("Genauigkeit (6)")) -> (F-format string=w402:string)  [unwired: 1 in]
              n137 = call <vilib>:"Space Constant.vi"() -> ("String"=w403:string)
              n138 = Search and Replace String(replace all?=TRUE ("Alle ersetzen? (F)"), input string=w402, search string=w403, replace string="0" ("Ersetzungs-String (\"\")")) -> (result string=w401:string)  [unwired: 4 in, 3 out]
              n139 = call "GD_MG_MagicFormula_OnOff.vi"("Aktion"=enum16{"lesen", "schreiben", "init"}."lesen") -> ("MG_use_magic_formula"=w389:bool)  [unwired: 8 in, 1 out]
              n140 = Build Array (concatenate)(w399, w387) -> (w391:dbl[])
              n141 = Build Array(w401) -> (w407:string[])
              n142 = call "GDC Kom.vi"("Befehl"=Aktion_Befehl."GD point", "Daten"=w407) -> ("Konzentration"=w393:string)  [unwired: 3 in, 6 out]
              n143 = Build Array (concatenate)(w398, w397) -> (w390:string[])
              n144 = Select(t=w385, s=w389, f=w388) -> (s? t:f=w384:dbl)
              n145 = call "GD_GesamtKonz_Teil_back_calc.vi"("Einheiten"=w390, "ohne Einheiten"=TRUE, "Konzentration der Komponenten"=w391, "Stufen"=w393, "Gesamtkonzentration"=w384, "Zeile"=w392, "Stufen Tabellen in (Eingang)"=w395) -> ("Stufen Tabellen in (Ausgang)"=w394:string[][][])  [unwired: 4 in]
            }
            frame #1 {
              n146 = call "GDC Kom.vi"("Befehl"=Aktion_Befehl."Standby") -> ()  [unwired: 4 in, 7 out]
            }
          }
        }
        frame 4, Default {
          # "HovaCAL, Horiba 710 c"
          n147 = Index Array(array=w418, index=w417) -> (element=w413:dbl)
          n148 = Build Array (concatenate)(w427, w418) -> (w421:dbl[])
          n149 = call "GD_MG_MagicFormula_OnOff.vi"("Aktion"=enum16{"lesen", "schreiben", "init"}."lesen") -> ("MG_use_magic_formula"=w414:bool)  [unwired: 8 in, 1 out]
          n150 = Unbundle By Name(w431) -> ("Gasteiler Stufen"=w430:T25)
          n151 = Build Array (concatenate)(w426, w425) -> (w420:string[])
          n152 = Select(t=w416, s=w414, f=w413) -> (s? t:f=w415:dbl)
          n153 = Index Array(array=w434, index (dim 0)=w417, index (dim 2)=0 ("Deaktivierter Index (Spalte)")) -> (element=w423:string[])  [unwired: 1 in]
          n154 = Fract/Exp String To Number(use system decimal point (T)=FALSE ("Systemdezimalzeichen verwenden (T)"), string=w423) -> (number=w432:dbl[])  [unwired: 2 in, 1 out]
          n155 = for {
            tunnel: w432 -> [w440] mode=indexing
            tunnel: w430 -> [w441]
            tunnel: w415 -> [w439]
            tunnel: [w435] -> w429 mode=indexing
            n156 = call "Mischverhaeltnis.vi"("Konzentration"=w440, "Sollwert"=w441) -> ("%"=w436:dbl)  [unwired: 8 in, 1 out]
            n157 = Divide(x=w439, y=sgl 100.0) -> (x/y=w437:dbl)
            n158 = Multiply(x=w436, y=w437) -> (x*y=w435:dbl)
          }
          n159 = Number To Fractional String(number=w429, precision (6)=i16 2 ("Genauigkeit (6)")) -> (F-format string=w422:string[])  [unwired: 2 in]
          n160 = call "GD_GesamtKonz_back_calc.vi"("Gesamtkonzentration"=w415, "Einheiten"=w420, "Konzentration der Komponenten"=w421, "Stufen"=w422, "Punkte (Eingang)"=w423) -> ("Stufentabellen (Ausgang)"=w419:string[][][])  [unwired: 5 in, 1 out]
        }
        frame 500 {
          # "Horiba 710 c ... manuell !"
        }
      }
    }
    frame True {
    }
  }
  n161 = Bundle By Name(cluster=T5 {"Stufen Tabellen out"=[], "EGAK"=[], "AGAK"=[]} ("GD out"), "Stufen Tabellen out"=w49, "EGAK"=w48) -> (→"GD out":T5)
  n162 = Decrement(x=w3) -> (x-1=→"Component Index out":i32)
  "error out" <- "error in (no error)"
